vi "Regularisation.vi"(6 "W":dbl[](array[numeric]), 8 "tau_f":dbl=15.0 format="%#_13g", 9 "Phi":dbl[](array[numeric]), 10 "Forgetting?":bool, 11 "dt":dbl) -> (3 "Forgetting Term":dbl[](array[numeric]))   [LabVIEW 2021]
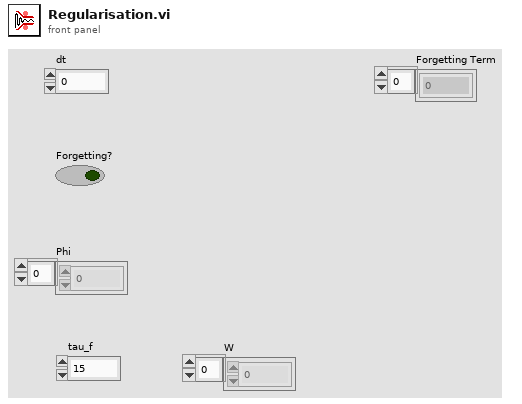
[diagram p1: front panel]
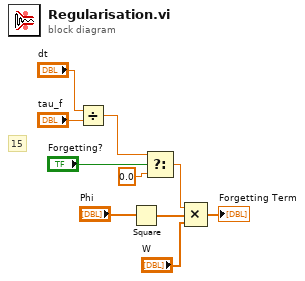
[diagram p0: block diagram]
diagram:
  # "15"
  n1 = Divide(x="dt", y="tau_f") -> (x/y=w4:dbl)
  n2 = Square(x="Phi") -> (x^2=w6:dbl[])
  n3 = Select(t=w4, s="Forgetting?", f=0.0) -> (s? t:f=w7:dbl)
  n4 = Compound Arithmetic op=MULTIPLY(w7, w6, "W") -> (→"Forgetting Term":dbl[])
